vi "Copy Result To Clipboard.vi"(0 "No. Of Decimal Places (6)":u32=6 step=1, 1 "Input":dbl step=0.1 format="%.6f") -> ()   [LabVIEW 2026]
doc: "This VI takes a floating-point number between 0 and 1 and maps it to another floating-point number between 0 and 1."
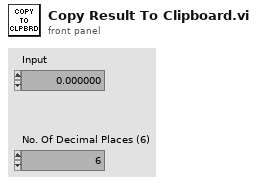
[diagram p1: front panel]
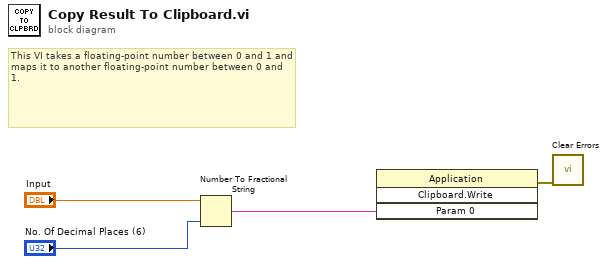
[diagram p0: block diagram]
diagram:
  # "This VI takes a floating-point number between 0 and 1 and maps it to another floating-point number between 0 and 1."
  n1 = Number To Fractional String(number="Input", precision (6)="No. Of Decimal Places (6)") -> (F-format string=w2:string)  [unwired: 2 in]
  n2 = invoke class="Application" method="Clipboard.Write"("Param 0"=w2) -> (error out=w1:errorcluster)  [unwired: 3 in, 3 out]
  n3 = call <vilib>:"Clear Errors.vi"("error in (no error)"=w1) -> ()  [unwired: 5 in, 2 out]
